vi "Main - GERM.vi"() -> ()   [LabVIEW 2023]
uses:
  <vilib>/addons/VeriStand Custom Device Scripting APIs/Data Sharing Framework/DSF Core.lvlibp/Typedefs/DSF Engine Framework Configuration.ctl
  <vilib>/addons/VeriStand Custom Device Scripting APIs/Data Sharing Framework/DSF Core.lvlibp/Typedefs/DSF Engine Plugin Configuration.ctl
  <vilib>/addons/VeriStand Custom Device Scripting APIs/Data Sharing Framework/DSF Core.lvlibp/Typedefs/Core Plugin Configuration.ctl
  <vilib>/addons/VeriStand Custom Device Scripting APIs/Data Sharing Framework/DSF Core.lvlibp/Typedefs/DSF Timing Info.ctl
  <vilib>/addons/VeriStand Custom Device Scripting APIs/Data Sharing Framework/DSF Core.lvlibp/Typedefs/DSF Settings Info.ctl
  <vilib>/addons/VeriStand Custom Device Scripting APIs/Data Sharing Framework/DSF Core.lvlibp/Typedefs/DSF Engine Plugin Thread Configuration.ctl
  <vilib>/addons/VeriStand Custom Device Scripting APIs/Data Sharing Framework/DSF Core.lvlibp/Typedefs/Core Thread Configuration.ctl
  <vilib>/addons/VeriStand Custom Device Scripting APIs/Data Sharing Framework/DSF Core.lvlibp/Typedefs/DSF Engine Transfer Group Configuration.ctl
  <vilib>/addons/VeriStand Custom Device Scripting APIs/Data Sharing Framework/DSF Core.lvlibp/Typedefs/Core Group Configuration.ctl
  <vilib>/addons/VeriStand Custom Device Scripting APIs/Data Sharing Framework/DSF Core.lvlibp/Typedefs/DSF Direction.ctl
  <vilib>/addons/VeriStand Custom Device Scripting APIs/Data Sharing Framework/DSF Core.lvlibp/Typedefs/DSF Timeout Behavior.ctl
  <vilib>/addons/VeriStand Custom Device Scripting APIs/Data Sharing Framework/DSF Core.lvlibp/Typedefs/DSF Engine Transfer Configuration.ctl
  <vilib>/addons/VeriStand Custom Device Scripting APIs/Data Sharing Framework/DSF Core.lvlibp/Typedefs/Core Transfer Configuration.ctl
  <vilib>/addons/VeriStand Custom Device Scripting APIs/Data Sharing Framework/DSF Core.lvlibp/Typedefs/DSF Engine Channel Configuration.ctl
  <vilib>/addons/VeriStand Custom Device Scripting APIs/Data Sharing Framework/DSF Core.lvlibp/Typedefs/Core Channel Configuration.ctl
  <vilib>/addons/VeriStand Custom Device Scripting APIs/Data Sharing Framework/DSF Core.lvlibp/Typedefs/DSF Data Type.ctl
  <userlib>/_OpenG.lib/array/array.llb/Index 1D Array Elements (String)__ogtk.vi
  <userlib>/_OpenG.lib/array/array.llb/Remove Duplicates from 1D Array (String)__ogtk.vi
  <userlib>/_OpenG.lib/array/array.llb/Filter 1D Array with Scalar (String)__ogtk.vi
  <vilib>/addons/VeriStand Custom Device Scripting APIs/Data Sharing Framework/DSF Core.lvlibp
  <vilib>/addons/VeriStand Custom Device Scripting APIs/Data Sharing Framework/DSF Core.lvlibp/Classes/Configuration/Core/Channel/Channel Configuration.lvclass
  <userlib>/_OpenG.lib/array/array.llb/openg_array.lvlib
  <vilib>/addons/VeriStand Custom Device Scripting APIs/Data Sharing Framework/DSF Core.lvlibp/Classes/Configuration/Core/Plugin/Plugin Configuration.lvclass
  <vilib>/addons/VeriStand Custom Device Scripting APIs/Data Sharing Framework/DSF Core.lvlibp/Classes/Configuration/Core/Thread/Thread Configuration.lvclass
  <vilib>/addons/VeriStand Custom Device Scripting APIs/Data Sharing Framework/DSF Core.lvlibp/Classes/Configuration/Core/Group/Group Configuration.lvclass
  <vilib>/addons/VeriStand Custom Device Scripting APIs/Data Sharing Framework/DSF Core.lvlibp/Classes/Configuration/Core/Transfer/Transfer Configuration.lvclass
panel:
  in  "Tab Control":enum32{"Main", "Raw Data", "Raw JSON"}(tab)
  out "DSF Clusters":T1[](array[typedef])
  out "Target Sources":string[](array[string])
  out "Channel Names":string[](array[string])
  out "Channel Units":string[](array[string])
  out "Channel Types":string[](array[string])
  out "Target Destinations":string[][](array[string])
  out "JSON Strings":string[](array[string])
  out "VISA Resource Names":string[](array[string])
  out "Target Names":string[](array[string])
  in  "File Path Control":path
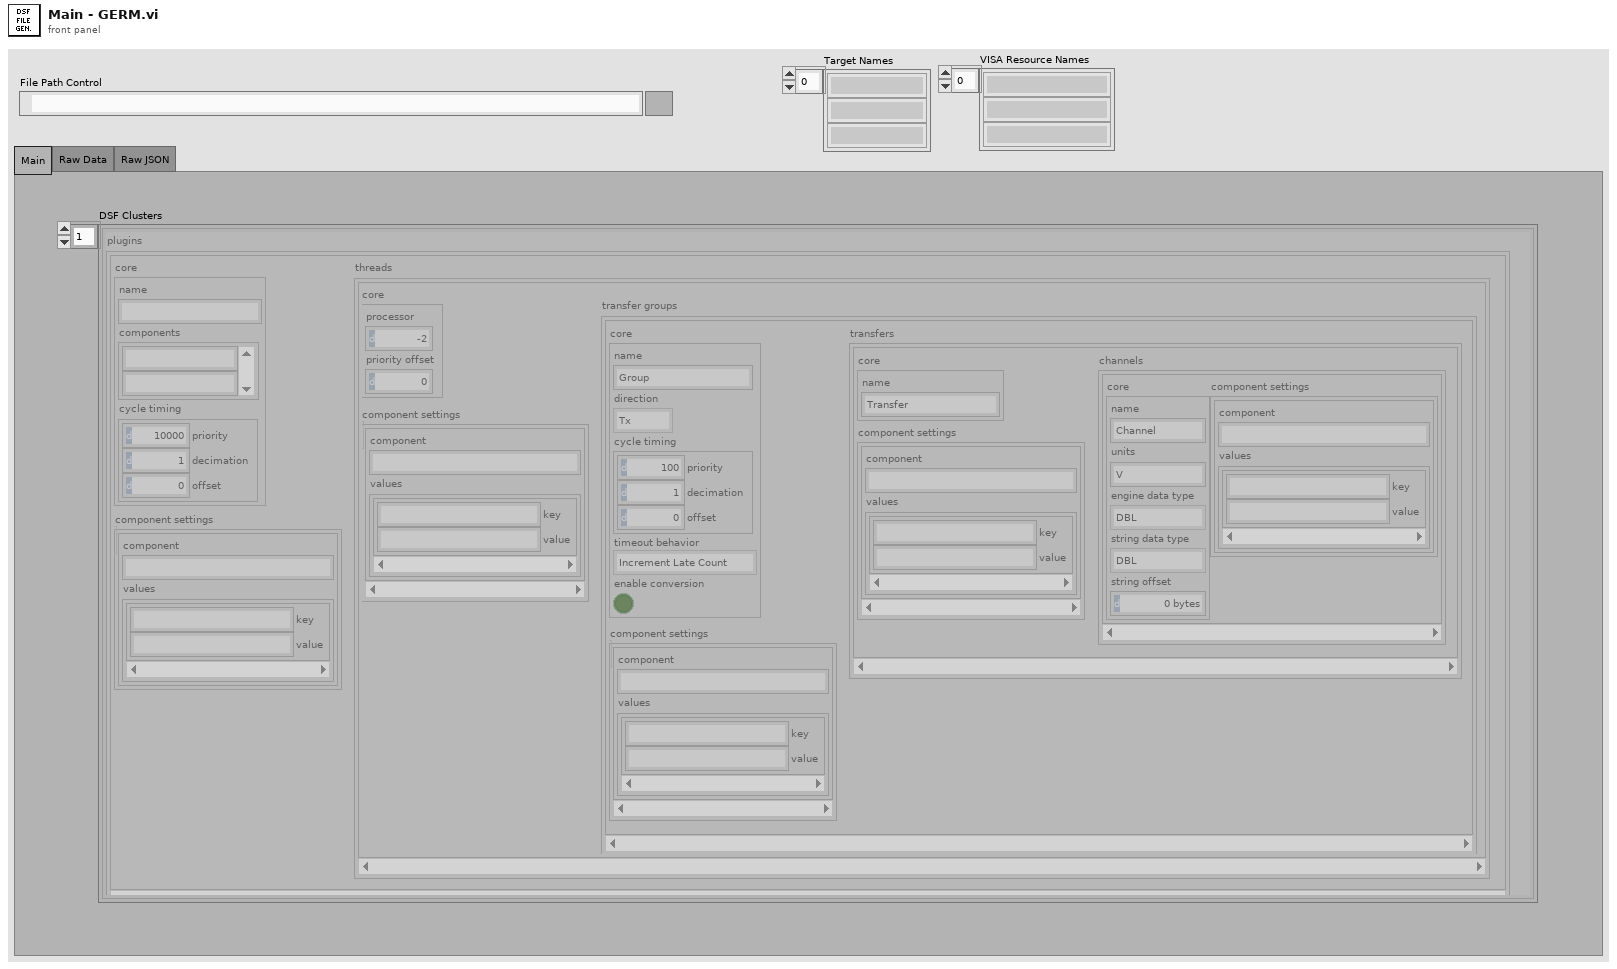
[diagram p1: front panel]
types:
  T1 = typedef "DSF Core.lvlibp/DSF Engine Framework Configuration.ctl" = cluster{"plugins":T2[]}
  T2 = typedef "DSF Core.lvlibp/DSF Engine Plugin Configuration.ctl" = cluster{"core":T3, "component settings":T5[], "threads":T6[]}
  T3 = typedef "DSF Core.lvlibp/Plugin Configuration.lvclass/Core Plugin Configuration.ctl" = cluster{"name":string, "components":string[], "cycle timing":T4}
  T4 = typedef "DSF Core.lvlibp/DSF Timing Info.ctl" = cluster{"priority":u64, "decimation":u64, "offset":u64}
  T5 = typedef "DSF Core.lvlibp/DSF Settings Info.ctl" = cluster{"component":string, "values":cluster{"key":string, "value":string}[]}
  T6 = typedef "DSF Core.lvlibp/DSF Engine Plugin Thread Configuration.ctl" = cluster{"core":T7, "component settings":T5[], "transfer groups":T8[]}
  T7 = typedef "DSF Core.lvlibp/Thread Configuration.lvclass/Core Thread Configuration.ctl" = cluster{"processor":i32, "priority offset":i16}
  T8 = typedef "DSF Core.lvlibp/DSF Engine Transfer Group Configuration.ctl" = cluster{"core":T9, "component settings":T5[], "transfers":T12[]}
  T9 = typedef "DSF Core.lvlibp/Group Configuration.lvclass/Core Group Configuration.ctl" = cluster{"name":string, "direction":T10, "cycle timing":T4, "timeout behavior":T11, "enable conversion":bool}
  T10 = typedef "DSF Core.lvlibp/DSF Direction.ctl" = enum8{"Tx", "Rx"}
  T11 = typedef "DSF Core.lvlibp/DSF Timeout Behavior.ctl" = enum8{"Increment Late Count", "Throw Error"}
  T12 = typedef "DSF Core.lvlibp/DSF Engine Transfer Configuration.ctl" = cluster{"core":T13, "component settings":T5[], "channels":T14[]}
  T13 = typedef "DSF Core.lvlibp/Transfer Configuration.lvclass/Core Transfer Configuration.ctl" = cluster{"name":string}
  T14 = typedef "DSF Core.lvlibp/DSF Engine Channel Configuration.ctl" = cluster{"core":T15, "component settings":T5[]}
  T15 = typedef "DSF Core.lvlibp/Channel Configuration.lvclass/Core Channel Configuration.ctl" = cluster{"name":string, "units":string, "engine data type":T16, "string data type":T16, "string offset":u64}
  T16 = typedef "DSF Core.lvlibp/DSF Data Type.ctl" = enum8{"Bool", "SGL", "DBL", "I8", "I16", "I32", "I64", "U8", "U16", "U32", "U64"}
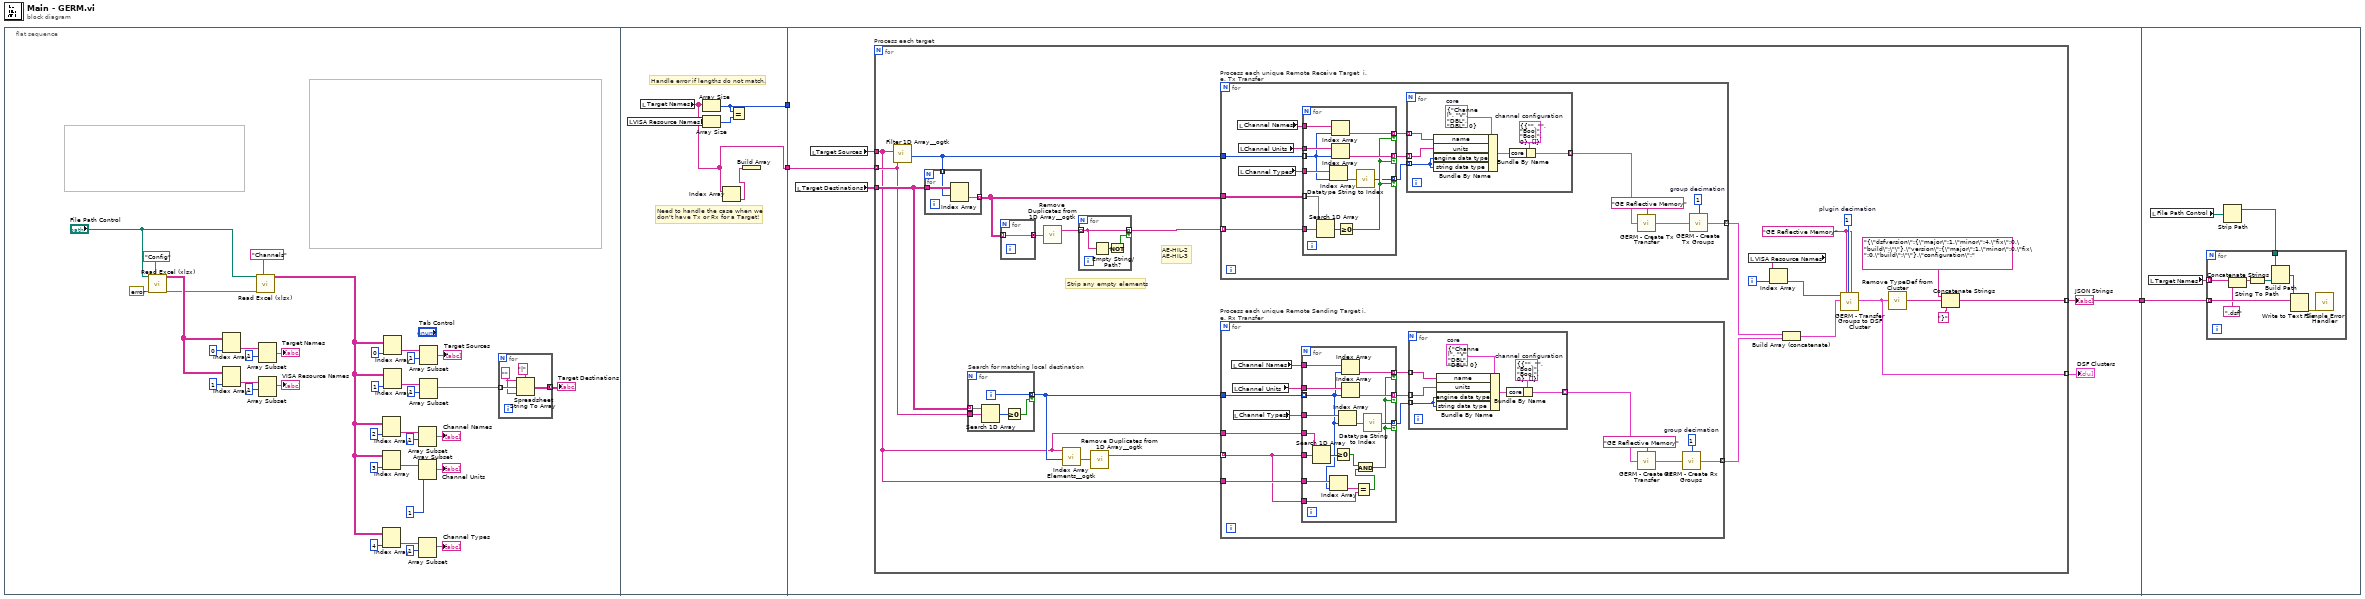
[diagram p0: block diagram]
diagram:
  n1 = flat-sequence {
    tunnel: [w47] -> w3
    tunnel: [w44] -> w1
    tunnel: w3 -> [_]
    tunnel: [w49] -> w2
    tunnel: w1 -> [w53]
    tunnel: w2 -> [w164]
    frame #0 {
      n2 = call "Read Excel (xlsx).vi"("Excel._SheetName"="Config", "error in (no error)"=errorcluster {"status"=FALSE, "code"=0, "source"=""}, "File Path Control"="File Path Control") -> ("error out"=w9:errorcluster, "data"=w10:string[][])  [unwired: 7 in]
      n3 = Index Array(array=w10, index (col)=0 ("disabled index (col)")) -> (element=w37:string[])  [unwired: 1 in]
      n4 = Index Array(array=w10, index (col)=1 ("disabled index (col)")) -> (element=w33:string[])  [unwired: 1 in]
      n5 = call "Read Excel (xlsx).vi"("Excel._SheetName"="Channels", "error in (no error)"=w9, "File Path Control"="File Path Control") -> ("data"=w8:string[][])  [unwired: 7 in, 1 out]
      n6 = Array Subset(array=w37, index=1) -> (→"Target Names":string[])  [unwired: 1 in]
      n7 = Array Subset(array=w33, index=1) -> (→"VISA Resource Names":string[])  [unwired: 1 in]
      n8 = Index Array(array=w8, index (col)=2 ("disabled index (col)")) -> (element=w22:string[])  [unwired: 1 in]
      n9 = Index Array(array=w8, index (col)=3 ("disabled index (col)")) -> (element=w18:string[])  [unwired: 1 in]
      n10 = Index Array(array=w8, index (col)=4 ("disabled index (col)")) -> (element=w14:string[])  [unwired: 1 in]
      n11 = Index Array(array=w8, index (col)=0 ("disabled index (col)")) -> (element=w29:string[])  [unwired: 1 in]
      n12 = Index Array(array=w8, index (col)=1 ("disabled index (col)")) -> (element=w25:string[])  [unwired: 1 in]
      n13 = Array Subset(array=w22, index=1) -> (→"Channel Names":string[])  [unwired: 1 in]
      n14 = Array Subset(array=w18, index=1) -> (→"Channel Units":string[])  [unwired: 1 in]
      n15 = Array Subset(array=w14, index=1) -> (→"Channel Types":string[])  [unwired: 1 in]
      n16 = Array Subset(array=w29, index=1) -> (→"Target Sources":string[])  [unwired: 1 in]
      n17 = Array Subset(array=w25, index=1) -> (w5:string[])  [unwired: 1 in]
      n18 = for {
        tunnel: w5 -> [w43] mode=indexing
        tunnel: [w41] -> w4 mode=concatenating
        w40 = ""
        n19 = Spreadsheet String To Array(delimiter (Tab)="|", format string=w40, spreadsheet string=w43, array type (2D Dbl)=w40) -> (array=w41:string[][])
      }
      "Target Destinations" <- w4
    }
    frame #1 {
      # "Need to handle the case when we \ndon't have Tx or Rx for a Target!"
      # "Handle error if lengths do not match."
      n20 = local read "VISA Resource Names"() -> (w46:string[])
      n21 = local read "Target Names"() -> (w44:string[])
      n22 = Array Size(array=w44) -> (size(s)=w47:i32)
      n23 = Array Size(array=w46) -> (size(s)=w48:i32)
      n24 = Index Array(array=w44) -> (element=w45:string)  [unwired: 1 in]
      n25 = Equal?(x=w47, y=w48) -> ()  [unwired: 1 out]
      n26 = Build Array(w45) -> ()  [unwired: 1 out]
    }
    frame #2 {
      n27 = local read "Target Destinations"() -> (w51:string[][])
      n28 = local read "Target Sources"() -> (w52:string[])
      n29 = for "Process each target" {
        tunnel: w53 -> [w63] mode=indexing
        tunnel: w52 -> [w62]
        tunnel: w51 -> [w71]
        tunnel: [w66] -> w49 mode=indexing
        tunnel: [w65] -> w50 mode=indexing
        i -> [w54]
        w57 = "GE Reflective Memory" ("plugin name")
        w58 = u64 1  # plugin decimation
        # "AE-HIL-2\nAE-HIL-3"
        # "Strip any empty elements"
        n30 = call-poly <userlib>:"Filter 1D Array__ogtk.vi"("items to filter"=w63, "array"=w62) -> ("filtered item indices"=w74:i32[])  [unwired: 4 in, 1 out]
        n31 = for {
          tunnel: w74 -> [w160] mode=indexing
          tunnel: w71 -> [w161]
          tunnel: [w159] -> w73 mode=indexing
          n32 = Index Array(array=w161, index (row)=w160) -> (element=w159:string[])  [unwired: 1 in]
        }
        n33 = for "Search for matching local destination" {
          tunnel: w71 -> [w121] mode=indexing
          tunnel: w63 -> [w120]
          tunnel: [w118] -> w70 mode=indexing if=w117
          i -> [w118]
          n34 = Search 1D Array(1D array=w121, element=w120) -> (index of element=w119:i32)  [unwired: 1 in]
          n35 = Greater Or Equal To 0?(x=w119) -> (x >= 0?=w117:bool)
        }
        n36 = for {
          tunnel: w73 -> [w158] mode=indexing
          tunnel: [w158] -> w77 mode=concatenating
        }
        n37 = call-poly <userlib>:"Remove Duplicates from 1D Array__ogtk.vi"("Input Array"=w77) -> ("Output Array"=w76:string[])  [unwired: 1 out]
        n38 = call-poly <userlib>:"Index Array Elements__ogtk.vi"("indices"=w70, "array"=w62) -> ("elements"=w72:string[])  [unwired: 9 in]
        n39 = for {
          tunnel: w76 -> [w157] mode=indexing
          tunnel: [w157] -> w75 mode=indexing if=w155
          n40 = Empty String/Path?(string/path=w157) -> (empty?=w156:bool)
          n41 = Not(x=w156) -> (.not. x?=w155:bool)
        }
        n42 = call-poly <userlib>:"Remove Duplicates from 1D Array__ogtk.vi"("Input Array"=w72) -> ("Output Array"=w64:string[])  [unwired: 1 out]
        n43 = for "Process each unique Remote Receive Target  i.e. Tx Transfer" {
          tunnel: w75 -> [w128] mode=indexing
          tunnel: w74 -> [w135]
          tunnel: w73 -> [w134]
          tunnel: [w124] -> w61 mode=indexing
          w123 = u64 1  # group decimation
          n44 = local read "Channel Names"() -> (w133:string[])
          n45 = local read "Channel Units"() -> (w132:string[])
          n46 = local read "Channel Types"() -> (w127:string[])
          n47 = for {
            tunnel: w134 -> [w154] mode=indexing
            tunnel: w128 -> [w153]
            tunnel: w135 -> [w146] mode=indexing
            tunnel: w133 -> [w151]
            tunnel: w132 -> [w150]
            tunnel: [w149] -> w131 mode=indexing if=w145
            tunnel: [w148] -> w130 mode=indexing if=w145
            tunnel: w127 -> [w147]
            tunnel: [w143] -> w126 mode=indexing if=w145
            n48 = Search 1D Array(1D array=w154, element=w153) -> (index of element=w152:i32)  [unwired: 1 in]
            n49 = Index Array(array=w147, index=w146) -> (element=w144:string)
            n50 = Index Array(array=w151, index=w146) -> (element=w149:string)
            n51 = Index Array(array=w150, index=w146) -> (element=w148:string)
            n52 = Greater Or Equal To 0?(x=w152) -> (x >= 0?=w145:bool)
            n53 = call "Datatype String to Index.vi"("Datatype String"=w144) -> ("Datatype"=w143:T16)  [unwired: 14 in]
          }
          n54 = for {
            tunnel: w131 -> [w139] mode=indexing
            tunnel: w130 -> [w138] mode=indexing
            tunnel: [w137] -> w129 mode=indexing
            tunnel: w126 -> [w136] mode=indexing
            w140 = T15 {"name"="Channel", "units"="V", "engine data type"=enum."DBL", "string data type"=enum."DBL", "string offset"=0}  # core
            w141 = T14 {"core"={"name"="", "units"="", "engine data type"=enum."Bool", "string data type"=enum."Bool", "string offset"=0}, "component settings"=[]}  # channel configuration
            n55 = Bundle By Name(cluster=w140, "name"=w139, "units"=w138, "engine data type"=w136, "string data type"=w136) -> (w142:T15)
            n56 = Bundle By Name(cluster=w141, "core"=w142) -> (w137:T14)
          }
          n57 = call "GERM - Create Tx Transfer.vi"("component name"="GE Reflective Memory", "tx channels"=w129) -> ("Transfer"=w125:T12)  [unwired: 13 in]
          n58 = call "GERM - Create Tx Groups.vi"("group decimation"=w123, "Tx Transfers"=w125) -> ("Tx Transfer Group"=w124:T8)  [unwired: 13 in]
        }
        n59 = for "Process each unique Remote Sending Target i.e. Rx Transfer" {
          tunnel: w64 -> [w84] mode=indexing
          tunnel: w70 -> [w92]
          tunnel: w62 -> [w91]
          tunnel: w62 -> [w85]
          tunnel: [w81] -> w60 mode=indexing
          w79 = u64 1  # group decimation
          n60 = local read "Channel Names"() -> (w90:string[])
          n61 = local read "Channel Units"() -> (w89:string[])
          n62 = local read "Channel Types"() -> (w82:string[])
          n63 = for {
            tunnel: w84 -> [w115]
            tunnel: w92 -> [w100] mode=indexing
            tunnel: w91 -> [w104]
            tunnel: w90 -> [w114]
            tunnel: w89 -> [w113]
            tunnel: [w112] -> w88 mode=indexing if=w102
            tunnel: [w111] -> w87 mode=indexing if=w102
            tunnel: w85 -> [w110]
            tunnel: w84 -> [w108]
            tunnel: [w103] -> w83 mode=indexing if=w102
            tunnel: w82 -> [w101]
            n64 = Search 1D Array(1D array=w104, element=w115) -> (index of element=w116:i32)  [unwired: 1 in]
            n65 = Index Array(array=w110, index=w100) -> (element=w109:string)
            n66 = Greater Or Equal To 0?(x=w116) -> (x >= 0?=w107:bool)
            n67 = Index Array(array=w101, index=w100) -> (element=w105:string)
            n68 = Index Array(array=w114, index=w100) -> (element=w112:string)
            n69 = Index Array(array=w113, index=w100) -> (element=w111:string)
            n70 = Equal?(x=w109, y=w108) -> (x = y?=w106:bool)
            n71 = And(x=w107, y=w106) -> (x .and. y?=w102:bool)
            n72 = call "Datatype String to Index.vi"("Datatype String"=w105) -> ("Datatype"=w103:T16)  [unwired: 14 in]
          }
          n73 = for {
            tunnel: w88 -> [w96] mode=indexing
            tunnel: w87 -> [w95] mode=indexing
            tunnel: [w94] -> w86 mode=indexing
            tunnel: w83 -> [w93] mode=indexing
            w97 = T15 {"name"="Channel", "units"="V", "engine data type"=enum."DBL", "string data type"=enum."DBL", "string offset"=0}  # core
            w98 = T14 {"core"={"name"="", "units"="", "engine data type"=enum."Bool", "string data type"=enum."Bool", "string offset"=0}, "component settings"=[]}  # channel configuration
            n74 = Bundle By Name(cluster=w97, "name"=w96, "units"=w95, "engine data type"=w93, "string data type"=w93) -> (w99:T15)
            n75 = Bundle By Name(cluster=w98, "core"=w99) -> (w94:T14)
          }
          n76 = call "GERM - Create Rx Transfer.vi"("component name"="GE Reflective Memory", "rx channels"=w86) -> ("Transfer"=w80:T12)  [unwired: 13 in]
          n77 = call "GERM - Create Rx Groups.vi"("group decimation"=w79, "Rx Transfers"=w80) -> ("Rx Transfer Group"=w81:T8)  [unwired: 13 in]
        }
        n78 = local read "VISA Resource Names"() -> (w56:string[])
        n79 = Index Array(array=w56, index=w54) -> (element=w55:string)
        n80 = Build Array (concatenate)(w61, w60) -> (w59:T8[])
        n81 = call "GERM - Transfer Groups to DSF Cluster.vi"("visa resource"=w55, "Transfer Groups"=w59, "plugin name"=w57, "plugin decimation"=w58, "component name"=w57) -> ("DSF Cluster"=w65:T1)  [unwired: 14 in]
        n82 = call "Remove TypeDef from Cluster.vi"("configuration 1.4"=w65) -> ("JSON string"=w69:string)  [unwired: 14 in]
        n83 = Concatenate Strings("{\"dsfversion\":{\"major\":1,\"minor\":4,\"fix\":0,\"build\":\"\"},\"version\":{\"major\":1,\"minor\":0,\"fix\":0,\"build\":\"\"},\"configuration\":", w69, "}") -> (w66:string)
      }
      "JSON Strings" <- w49
      "DSF Clusters" <- w50
    }
    frame #3 {
      n84 = local read "Target Names"() -> (w163:string[])
      n85 = local read "File Path Control"() -> (w165:path)
      n86 = Strip Path(path=w165) -> (stripped path=w162:path)  [unwired: 1 out]
      n87 = for {
        tunnel: w164 -> [w173] mode=indexing
        tunnel: w163 -> [w169] mode=indexing
        tunnel: w162 -> [w172]
        n88 = Concatenate Strings(w169, ".dsf" ("string")) -> (w168:string)
        n89 = String To Path(string=w168) -> (path=w171:path)
        n90 = Build Path(base path=w172, name or relative path=w171) -> (appended path=w170:path)
        n91 = Write to Text File(file (use dialog)=w170, text=w173) -> (error out=w166:errorcluster)  [unwired: 2 in, 2 out]
        n92 = call <vilib>:"Simple Error Handler.vi"("error in (no error)"=w166) -> ()  [unwired: 4 in, 5 out]
      }
    }
  }
